vi "Assign String Values.vi"(8 "error in (no error)":errorcluster, 9 "Arguments":string[](array[string]), 11 "LV Argument Parser in":refnum<class "LV Argument Parser.lvclass">) -> (0 "error IO":errorcluster, 3 "LV Argument Parser out":refnum<class "LV Argument Parser.lvclass">)   [LabVIEW 2023, in "LV ArgParse.lvlib" / "LV Argument Parser.lvclass"]
uses:
  LV Argument Parser.lvclass
  LV Argument Parser.lvclass/LV Argument Parser.ctl
  <vilib>/Utility/miscctls.llb/LVMapReplaceAction.ctl
  <vilib>/Utility/error.llb/Trim Whitespace One-Sided.vi
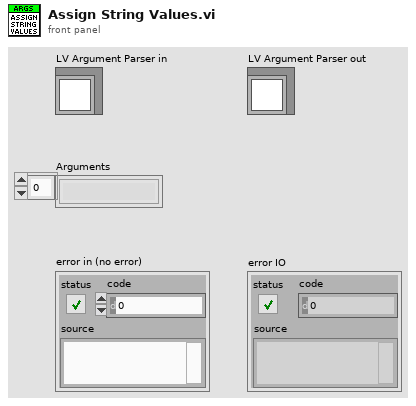
[diagram p1: front panel]
types:
  T1 = typedef "LVMapReplaceAction.ctl" = enum32{"Modify Entry only if found", "Add or Modify Entry", "Delete Entry"}
  T2 = typedef "LV ArgParse.lvlib/LV Argument Parser.lvclass/Argument Definition.ctl" = cluster{"Name":string, "short (positional)":string, "long (positional)":string, "action":enum16{"store", "store-const", "store-false", "store-true", "append", "append-const", "count", "help", "version"}, "choices":string[], "const":string, "default":string, "dest (=name)":string, "help":string, "Number":i32, "Required":bool, "Type":enum16{"String", "Int", "UInt", "Float", "Bool", "Date", "Path"}}
  T3 = enum16{"store", "store-const", "store-false", "store-true", "append", "append-const", "count", "help", "version"}
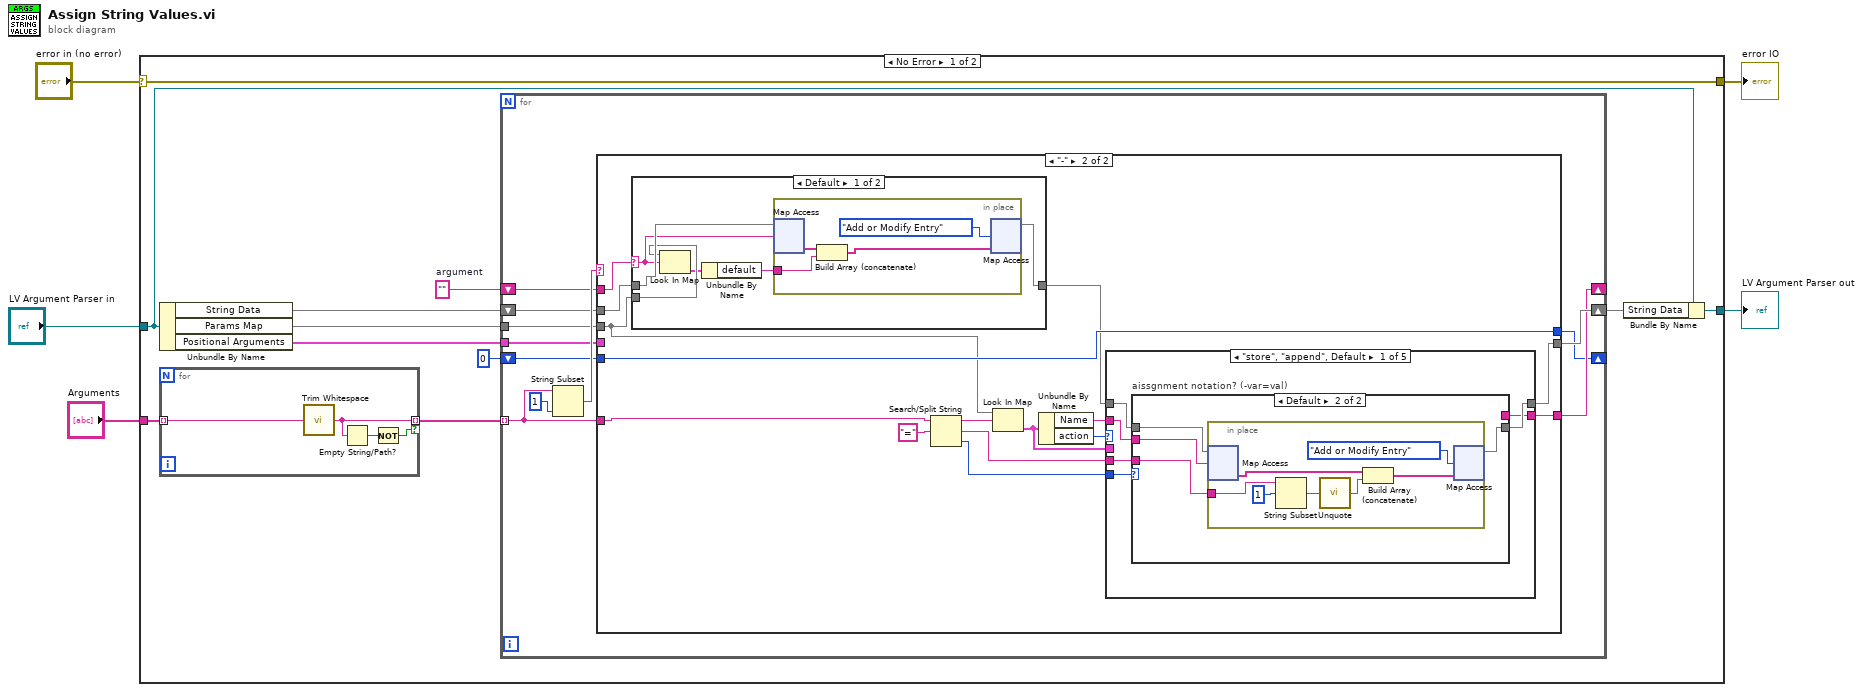
[diagram p0: block diagram]
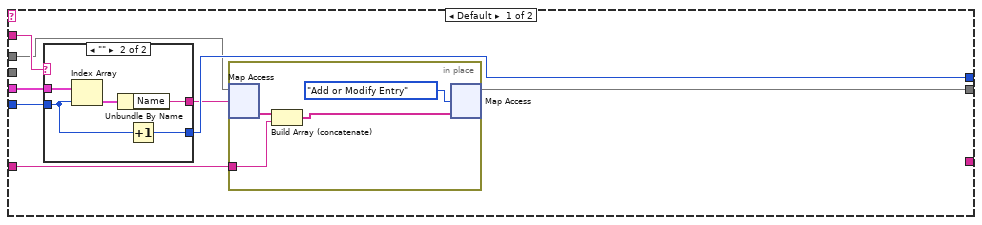
[diagram p2: hidden frame]
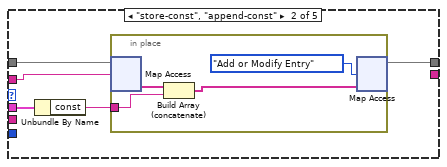
[diagram p6: hidden frame]
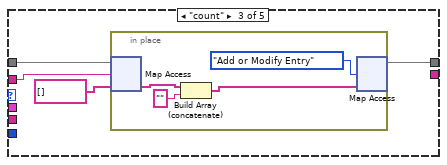
[diagram p7: hidden frame]
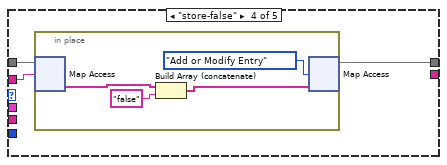
[diagram p8: hidden frame]
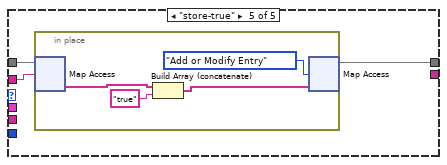
[diagram p9: hidden frame]
diagram:
  n1 = case shown="No Error" "error in (no error)" {
    selector: "error in (no error)" -> [w9 w128]
    tunnel: "LV Argument Parser in" -> [w13 w127]
    tunnel: [w11 w127] -> w4
    tunnel: [w9 w128] -> w2
    tunnel: "Arguments" -> [w8 _]
    frame No Error {
      w14 = ""  # argument
      n2 = Unbundle By Name(w13) -> ("String Data"=w6:map{string, string[]}, "Params Map"=w16:map{string, T2}, "Positional Arguments"=w10:T2[])
      n3 = for {
        tunnel: w8 -> [w20] mode=indexing
        tunnel: [w19] -> w7 mode=indexing if=w17
        n4 = call <vilib>:"Trim Whitespace.vi"("string"=w20) -> ("trimmed string"=w19:string)  [unwired: 1 in]
        n5 = Empty String/Path?(string/path=w19) -> (empty?=w18:bool)
        n6 = Not(x=w18) -> (.not. x?=w17:bool)
      }
      n7 = for {
        tunnel: w7 -> [w29] mode=indexing
        shift-right: [w28] -> w12
        shift-left: w6 -> [w27]
        shift-right: [w26] -> _
        shift-left: w14 -> [w25]
        tunnel: w10 -> [w24]
        shift-right: [w23] -> _
        shift-left: 0 -> [w22]
        tunnel: w16 -> [w21]
        n8 = String Subset(string=w29, length (rest)=1 ("length (rest)")) -> (substring=w30:string)  [unwired: 1 in]
        n9 = case shown="\"-\"" w30 {
          tunnel: w29 -> [w33 w55]
          tunnel: [w32 w62] -> w28
          tunnel: w27 -> [w35 w58]
          tunnel: [_ w63] -> w26
          tunnel: w25 -> [w39 w60]
          tunnel: w24 -> [w38 _]
          tunnel: [w37 w65] -> w23
          tunnel: w22 -> [w36 w65]
          tunnel: w21 -> [_ w57]
          frame Default {
            n10 = case shown="\"\"" w39 {
              selector: w39 -> [w44 _]
              tunnel: w38 -> [_ w50]
              tunnel: [w45 w48] -> w37
              tunnel: w36 -> [w45 w49]
              tunnel: [w44 w46] -> w34
              frame Default {
              }
              frame "" {
                n11 = Index Array(array=w50, index=w49) -> (element=w47:T2)
                n12 = Unbundle By Name(w47) -> ("Name"=w46:string)
                n13 = Increment(x=w49) -> (x+1=w48:i32)
              }
            }
            n14 = in-place {
              in-place-border: w33 -> [w41]
              n15 = in-place-map #1(w35, w34) -> (w43:string[])  [unwired: 1 in, 1 out]
              n16 = Build Array (concatenate)(w43, w41) -> (w42:string[])
              n17 = in-place-map #1(w42, LVMapReplaceAction."Add or Modify Entry" ("action")) -> (w32:map{string, string[]})  [unwired: 2 out]
            }
          }
          frame "-" {
            n18 = case shown="Default" w60 {
              selector: w60 -> [w67 _]
              tunnel: [w68 w76] -> w59
              tunnel: w58 -> [w71 w76]
              tunnel: w57 -> [w70 _]
              frame Default {
                n19 = Look In Map(map=w70, key=w67) -> (value=w69:T2)  [unwired: 1 in, 1 out]
                n20 = Unbundle By Name(w69) -> ("default"=w66:string)
                n21 = in-place {
                  in-place-border: w66 -> [w72]
                  n22 = in-place-map #2(w71, w67) -> (w75:string[])  [unwired: 1 in, 1 out]
                  n23 = Build Array (concatenate)(w75, w72) -> (w73:string[])
                  n24 = in-place-map #2(w73, LVMapReplaceAction."Add or Modify Entry" ("action")) -> (w68:map{string, string[]})  [unwired: 2 out]
                }
              }
              frame "" {
              }
            }
            n25 = Search/Split String(string=w55, search string/char (-)="=") -> (substring before match=w53:string, match + rest of string=w52:string, offset of match=w51:i32)  [unwired: 1 in]
            n26 = Look In Map(map=w57, key=w53) -> (value=w61:T2)  [unwired: 1 in, 1 out]
            n27 = Unbundle By Name(w61) -> ("Name"=w56:string, "action"=w64:T3)
            n28 = case shown="\"store\", \"append\", Default" w64 {
              tunnel: w61 -> [_ w100 _ _ _]
              tunnel: [w77 _ _ _ _] -> w63
              tunnel: w56 -> [w80 w97 w106 w113 w120]
              tunnel: [w81 w98 w107 w114 w121] -> w62
              tunnel: w59 -> [w82 w99 w108 w115 w122]
              tunnel: w52 -> [w79 _ _ _ _]
              tunnel: w51 -> [w78 _ _ _ _]
              frame "store", "append", Default {
                n29 = case "aissgnment notation? (-var=val)" shown="Default" w78 {
                  tunnel: w82 -> [w83 w88]
                  tunnel: [w83 w87] -> w81
                  tunnel: w80 -> [w84 w86]
                  tunnel: w79 -> [_ w85]
                  tunnel: [w84 _] -> w77
                  frame -1 {
                  }
                  frame Default {
                    n30 = in-place {
                      in-place-border: w85 -> [w92]
                      n31 = in-place-map #3(w88, w86) -> (w95:string[])  [unwired: 1 in, 1 out]
                      n32 = String Subset(string=w92, offset (0)=1) -> (substring=w90:string)  [unwired: 1 in]
                      n33 = call "Unquote.vi"("String"=w90) -> ("trimmed string"=w91:string)
                      n34 = Build Array (concatenate)(w95, w91) -> (w93:string[])
                      n35 = in-place-map #3(w93, LVMapReplaceAction."Add or Modify Entry" ("action")) -> (w87:map{string, string[]})  [unwired: 2 out]
                    }
                  }
                }
              }
              frame "store-const", "append-const" {
                n36 = Unbundle By Name(w100) -> ("const"=w96:string)
                n37 = in-place {
                  in-place-border: w96 -> [w102]
                  n38 = in-place-map #4(w99, w97) -> (w104:string[])  [unwired: 1 in, 1 out]
                  n39 = Build Array (concatenate)(w104, w102) -> (w103:string[])
                  n40 = in-place-map #4(w103, LVMapReplaceAction."Add or Modify Entry" ("action")) -> (w98:map{string, string[]})  [unwired: 2 out]
                }
              }
              frame "count" {
                n41 = in-place {
                  n42 = in-place-map #5(w108, w106, string[] []) -> (w112:string[])  [unwired: 1 out]
                  n43 = Build Array (concatenate)(w112, "") -> (w111:string[])
                  n44 = in-place-map #5(w111, LVMapReplaceAction."Add or Modify Entry" ("action")) -> (w107:map{string, string[]})  [unwired: 2 out]
                }
              }
              frame "store-false" {
                n45 = in-place {
                  n46 = in-place-map #6(w115, w113) -> (w119:string[])  [unwired: 1 in, 1 out]
                  n47 = Build Array (concatenate)(w119, "false" ("String")) -> (w118:string[])
                  n48 = in-place-map #6(w118, LVMapReplaceAction."Add or Modify Entry" ("action")) -> (w114:map{string, string[]})  [unwired: 2 out]
                }
              }
              frame "store-true" {
                n49 = in-place {
                  n50 = in-place-map #7(w122, w120) -> (w126:string[])  [unwired: 1 in, 1 out]
                  n51 = Build Array (concatenate)(w126, "true" ("String")) -> (w125:string[])
                  n52 = in-place-map #7(w125, LVMapReplaceAction."Add or Modify Entry" ("action")) -> (w121:map{string, string[]})  [unwired: 2 out]
                }
              }
            }
          }
        }
      }
      n53 = Bundle By Name(cluster=w13, "String Data"=w12) -> (w11:refnum<class "LV Argument Parser.lvclass">)
    }
    frame Error {
    }
  }
  "LV Argument Parser out" <- w4
  "error IO" <- w2
